vi "FPGA Server.vi"() -> ()   [LabVIEW 2014]
doc: "Accepts inputs from a host based VI for controlling analog and digital outputs on a R-series board containing an FPGA. This VI will produce 4 different signal types dependent on the user input and the channel of interest. When the <B>WaveType</B> is set to laser, the first three channels will produce either a sine or square wave at the frequency <B>f0</B> while the last two produce only square waves. When the wavetype is set to speaker or none, all channels produce the same signal (although for the speaker, signals with a gain of <B>Amp</B> applied)."
uses:
  Utilities/FPGA/Controls/FxdPt Props.ctl
  Reusable/PAS/Main/Controls/Laser Modulation.ctl
  <vilib>/Platform/TimedLoop/XDataNode/timing_clust.ctl
  <vilib>/Platform/TimedLoop/XDataNode/nitl_modes.ctl
  <vilib>/Platform/TimedLoop/XDataNode/wakeup.ctl
  <vilib>/rvi/Emulation/niFpgaGetClockAttributes.vi
  <vilib>/rvi/Emulation/niFpgaSctlEmulationGetInTimedLoop.vi
  <vilib>/rvi/Emulation/niFpgaEmulationReportErrorSimple.vi
  <vilib>/rvi/Emulation/niFpgaProcessEmulError.vi
  <vilib>/rvi/eio/common/nirviEmuTemplateMethod_errors.vi
  <vilib>/rvi/Memory/Memory_Emulation/nirvimemoryFastEmulation.vi
  <vilib>/rvi/Memory/Memory_Emulation/nirvimemoryEmulation.vi
  <vilib>/rvi/Emulation/niFpgaEmulationIsFPGAContextNoSignature.vi
  <vilib>/rvi/DataTransferAndStorage/Container/Common/niFpgaContainerGetUniqueNameForEmu.vi
  <vilib>/rvi/errors/nirviReportUnexpectedCaseInternalError (U32).vi
  <vilib>/rvi/Emulation/niFpgaCriticalErrorInLSC.vi
  <vilib>/rvi/interface/RandomDataEmulation/niFpgaRandomDataHandleErrors.vi
  <vilib>/eio/EIONode/EIONode.xnode
  <vilib>/rvi/DataTransferAndStorage/Container/XNode/niFpgaContainer.xnode
  <vilib>/rvi/FXPMathLib/FxpMul/XNode/nifxpmath_Multiplier.xnode
  <vilib>/rvi/FXPMathLib/FxpAdd/XNode/nifxpmath_Add.xnode
  <vilib>/rvi/interface/RandomDataEmulation/nirviRandomDataFpgaReadWriteTemplate.vi
  <vilib>/Platform/TimedLoop/XDataNode/XDataNode.xnode
  <vilib>/Platform/TimedLoop/XDataNode/XDNodeRunTimeDep.lvlib
  <vilib>/rvi/FXPMathLib/sim/FxpSim.dll
panel:
  out "Direction":bool
  out "error out":errorcluster
  in  "iSpk Enable":T1={"Ch1"=TRUE, "Ch2"=TRUE, "Ch3"=TRUE, "Ch4"=TRUE, "Ch5"=TRUE}
  in  "Speaker":cluster{"Voltage":fxp<+,14,1>, "Offset":i16}
  in  "Spk Enable":bool
  in  "LaserEn":T1
  in  "Cell 5":T2 {"Offset" format="%#.6f"; "Scale" format="%#.6f"}
  in  "Cell 4":T2 {"Offset" format="%#.6f"; "Scale" format="%#.6f"}
  in  "Cell 3":T2 {"Offset" format="%#.6f"; "Scale" format="%#.6f"}
  in  "Cell 2":T2 {"f0" format="%#.6g"; "Offset" format="%#.6f"; "Scale" format="%#.6f"}
  in  "Cell 1":T2 {"f0" format="%.0g"; "Offset" format="%#.6f"; "Scale" format="%#.6f"}
  out "Stopped":bool
  out "SquareOut":T4
  in  "stop":bool
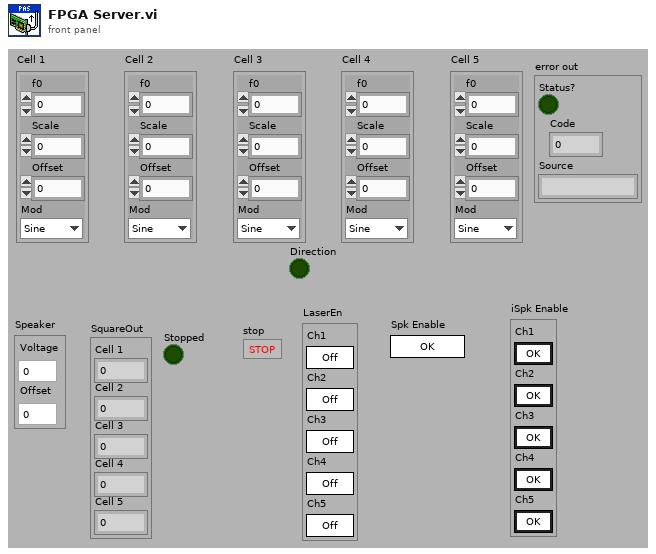
[diagram p1: front panel]
types:
  T1 = cluster{"Ch1":bool, "Ch2":bool, "Ch3":bool, "Ch4":bool, "Ch5":bool}
  T2 = typedef "FxdPt Props.ctl" = cluster{"f0":fxp<+,32,0>, "Scale":fxp<+,14,1>, "Offset":i16, "Mod":T3}
  T3 = typedef "Laser Modulation.ctl" = enum8{"Sine", "Square"}
  T4 = cluster{"Cell 1":i16, "Cell 2":i16, "Cell 3":i16, "Cell 4":i16, "Cell 5":i16}
  T5 = typedef "XDNodeRunTimeDep.lvlib/timing_clust.ctl" = cluster{"Expected End [f-1]":u64, "Actual End [f-1]":u64, "Finished Late? [f-1]":bool, "Expected End [i-1]":u64, "Actual End [i-1]":u64, "Finished Late? [i-1]":bool, "Expected Start [i]":u64, "Actual Start [i]":u64, "Expected Start [f]":u64, "Actual Start [f]":u64, "Source Name":string, "Structure Name":string, "Period":i64, "Deadline":i64, "Offset":i64, "Start":i64, "Priority":i32, "Timeout":i32, "Mode":T6, "Wakeup Reason":T7, "Error":errorcluster, "Source Type":string, "Secondary Source Type":string, "Global End Time":u64, "Global Start Time":u64, "Frame Duration":u64, "Iteration Duration":u64, "Assigned CPU":i32, "I/O Scan Engine Mode":u32}
  T6 = typedef "XDNodeRunTimeDep.lvlib/nitl_modes.ctl" = enum32{"No Change", "Process missed periods, maintain original phase", "Discard missed periods, maintain original phase", "Process missed periods, ignore original phase", "Discard missed periods, ignore original phase"}
  T7 = typedef "XDNodeRunTimeDep.lvlib/wakeup.ctl" = enum32{"Normal", "Aborted", "Asynchronous wakeup", "Timing source error", "Timed loop error", "Timeout"}
  T8 = cluster{"square wave out":i16, "square wave out":i16, "square wave out":i16, "square wave out":i16, "square wave out":i16}
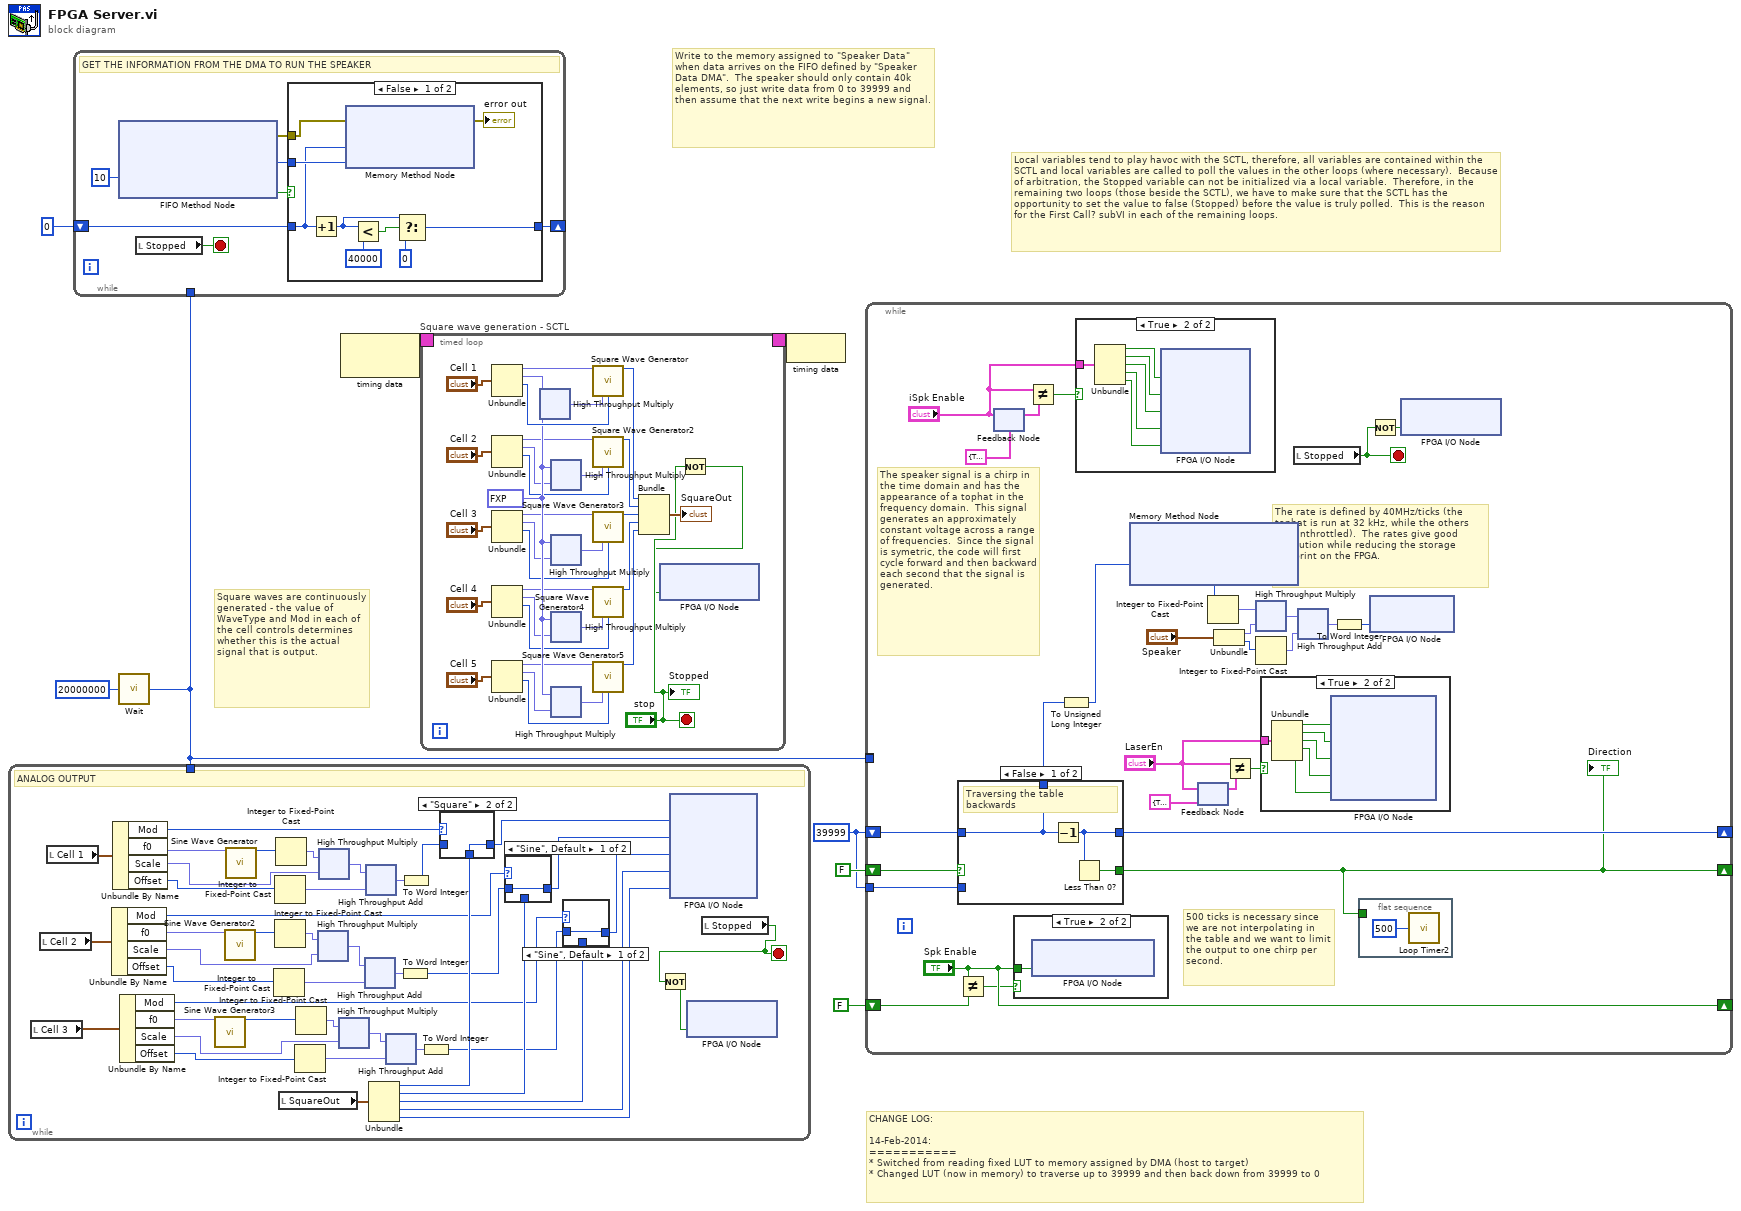
[diagram p0: block diagram]
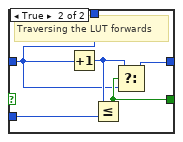
[diagram p6: hidden frame]
diagram:
  w3 = u32 20000000 ("Count(Ticks)")
  w1 = 39999
  # "Write to the memory assigned to \"Speaker Data\" when data arrives on the FIFO defined by \"Speaker Data DMA\".  The speaker should only contain 40k elements, so just write data from 0 to 39999 and then assume that the next write begins a new signal."
  # "CHANGE LOG:\n\n14-Feb-2014:\n===========\n* Switched from reading fixed LUT to memory assigned by DMA (host to target)\n* Changed LUT (now in memory) to traverse up to 39999 and then back down from 39999 to 0"
  # "Square waves are continuously generated - the value of WaveType and Mod in each of the cell controls determines whether this is the actual signal that is output."
  # "Local variables tend to play havoc with the SCTL, therefore, all variables are contained within the SCTL and local variables are called to poll the values in the other loops (where necessary).  Because of arbitration, the Stopped variable can not be initialized via a local variable.  Therefore, in the remaining two loops (those beside the SCTL), we have to make sure that the SCTL has the opportunity to set the value to false (Stopped) before the value is truly polled.  This is the reason for the First Call? subVI in each of the remaining loops."
  n1 = while "Analog Output" {
    tunnel: w3 -> [_]
    stop <- w9 stop-if-true
    # "ANALOG OUTPUT"
    n2 = local read "Cell 3"() -> (w16:T2)
    n3 = local read "Cell 2"() -> (w17:T2)
    n4 = local read "Cell 1"() -> (w18:T2)
    n5 = Unbundle By Name(w17) -> ("Mod"=w11:T3, "f0"=w29:fxp<+,32,0>, "Scale"=w28:fxp<+,14,1>, "Offset"=w27:i16)
    n6 = Unbundle By Name(w18) -> ("Mod"=w12:T3, "f0"=w37:fxp<+,32,0>, "Scale"=w36:fxp<+,14,1>, "Offset"=w35:i16)
    n7 = Unbundle By Name(w16) -> ("Mod"=w10:T3, "f0"=w24:fxp<+,32,0>, "Scale"=w25:fxp<+,14,1>, "Offset"=w26:i16)
    n8 = call "Sine Wave Generator3"("frequency (periods/tick)"=w24) -> ("sine out"=w21:i16)  [unwired: 14 in]
    n9 = call "Sine Wave Generator2"("frequency (periods/tick)"=w29) -> ("sine out"=w32:i16)  [unwired: 14 in]
    n10 = call "Sine Wave Generator"("frequency (periods/tick)"=w37) -> ("sine out"=w40:i16)  [unwired: 14 in]
    n11 = Integer to Fixed-Point Cast(integer=w27) -> (fixed-point=w34:fxp<+/-,16,16>)  [unwired: 1 in]
    n12 = Integer to Fixed-Point Cast(integer=w35) -> (fixed-point=w38:fxp<+/-,16,16>)  [unwired: 1 in]
    n13 = Integer to Fixed-Point Cast(integer=w32) -> (fixed-point=w33:fxp<+/-,16,16>)  [unwired: 1 in]
    n14 = Integer to Fixed-Point Cast(integer=w40) -> (fixed-point=w39:fxp<+/-,16,16>)  [unwired: 1 in]
    n15 = local read "SquareOut"() -> (w46:T4)
    n16 = Integer to Fixed-Point Cast(integer=w26) -> (fixed-point=w19:fxp<+/-,16,16>)  [unwired: 1 in]
    n17 = Integer to Fixed-Point Cast(integer=w21) -> (fixed-point=w20:fxp<+/-,16,16>)  [unwired: 1 in]
    n18 = xnode ("High Throughput Multiply")("x"=w33, "y"=w28) -> ("x*y"=w30:fxp<+/-,30,17>)
    n19 = xnode ("High Throughput Multiply")("x"=w39, "y"=w36) -> ("x*y"=w42:fxp<+/-,30,17>)
    n20 = xnode ("High Throughput Multiply")("x"=w20, "y"=w25) -> ("x*y"=w23:fxp<+/-,30,17>)
    n21 = xnode ("High Throughput Add")("x"=w30, "y"=w34) -> ("x+y"=w31:fxp<+/-,16,16>)
    n22 = xnode ("High Throughput Add")("x"=w42, "y"=w38) -> ("x+y"=w41:fxp<+/-,16,16>)
    n23 = Unbundle(w46) -> ("Cell 1"=w45:i16, "Cell 2"=w44:i16, "Cell 3"=w43:i16, "Cell 4"=w48:i16, "Cell 5"=w47:i16)
    n24 = xnode ("High Throughput Add")("x"=w23, "y"=w19) -> ("x+y"=w22:fxp<+/-,16,16>)
    n25 = To Word Integer(number=w31) -> (16bit integer=w14:i16)
    n26 = To Word Integer(number=w41) -> (16bit integer=w15:i16)
    n27 = To Word Integer(number=w22) -> (16bit integer=w13:i16)
    n28 = case shown="\"Square\"" w12 {
      tunnel: w45 -> [_ w57]
      tunnel: [w56 w57] -> w51
      tunnel: w15 -> [w56 _]
      frame "Sine", Default {
      }
      frame "Square" {
      }
    }
    n29 = case shown="\"Sine\", Default" w11 {
      tunnel: w44 -> [_ w55]
      tunnel: [w54 w55] -> w50
      tunnel: w14 -> [w54 _]
      frame "Sine", Default {
      }
      frame "Square" {
      }
    }
    n30 = case shown="\"Sine\", Default" w10 {
      tunnel: w43 -> [_ w53]
      tunnel: [w52 w53] -> w49
      tunnel: w13 -> [w52 _]
      frame "Sine", Default {
      }
      frame "Square" {
      }
    }
    n31 = xnode "FPGA I/O Node"("Ch 1 AO"=w51, "Ch 2 AO"=w50, "Ch 3 AO"=w49, "Ch 4 AO"=w48, "Ch 5 AO"=w47) -> ()  [unwired: 5 in, 5 out]
    n32 = local read "Stopped"() -> (w9:bool)
    n33 = Not(x=w9) -> (.not. x?=w8:bool)
    n34 = xnode "FPGA I/O Node"("AO Loop"=w8) -> ()  [unwired: 1 in, 1 out]
  }
  n35 = while {
    tunnel: w3 -> [_]
    shift-right: [w59] -> _
    shift-left: u32 0 ("Address") -> [w60]
    stop <- w64 stop-if-true
    # "GET THE INFORMATION FROM THE DMA TO RUN THE SPEAKER"
    n36 = xnode ("FIFO Method Node")("Timeout"=10) -> ("Element"=w62:i16, "Timed Out?"=w61:bool, "error out"=w58:errorcluster)  [unwired: 2 in, 1 out]
    n37 = local read "Stopped"() -> (w64:bool)
    n38 = case shown="False" w61 {
      tunnel: w62 -> [w73 _]
      tunnel: w60 -> [w72 w74]
      tunnel: [w67 w74] -> w59
      tunnel: w58 -> [w66 _]
      frame False {
        n39 = Increment(x=w72) -> (x+1=w69:u32)
        n40 = xnode ("Memory Method Node")("Address"=w72, "Data"=w73, "error in (no error)"=w66) -> ("error out"=→"error out":errorcluster)  [unwired: 1 in, 1 out]
        n41 = Less?(x=w69, y=u32 40000) -> (x < y?=w70:bool)
        n42 = Select(t=w69, s=w70, f=u32 0) -> (s? t:f=w67:u32)
      }
      frame True {
      }
    }
  }
  n43 = call "Wait"("Count(Ticks)"=w3) -> ()  [unwired: 1 out]
  n44 = node-c288() -> (w7:T5)  [unwired: 1 in]
  n45 = timed-loop "Square wave generation - SCTL" {
    timing: w7 -> [_]
    timing-out: [_] -> w6
    stop <- "stop" stop-if-true
    w97 = fxp<+,15,15> 32767.0 ("n")
    n46 = Unbundle("Cell 1") -> ("f0"=w100:fxp<+,32,0>, "Scale"=w99:fxp<+,14,1>, "Offset"=w98:i16)  [unwired: 1 out]
    n47 = Unbundle("Cell 2") -> ("f0"=w88:fxp<+,32,0>, "Scale"=w87:fxp<+,14,1>, "Offset"=w89:i16)  [unwired: 1 out]
    n48 = Unbundle("Cell 3") -> ("f0"=w85:fxp<+,32,0>, "Scale"=w86:fxp<+,14,1>, "Offset"=w90:i16)  [unwired: 1 out]
    n49 = Unbundle("Cell 4") -> ("f0"=w84:fxp<+,32,0>, "Scale"=w83:fxp<+,14,1>, "Offset"=w91:i16)  [unwired: 1 out]
    n50 = Unbundle("Cell 5") -> ("f0"=w78:fxp<+,32,0>, "Scale"=w77:fxp<+,14,1>, "Offset"=w92:i16)  [unwired: 1 out]
    n51 = xnode ("High Throughput Multiply")("x"=w99, "y"=w97) -> ("x*y"=w102:fxp<+,29,16>)
    n52 = xnode ("High Throughput Multiply")("x"=w97, "y"=w87) -> ("x*y"=w80:fxp<+,29,16>)
    n53 = xnode ("High Throughput Multiply")("x"=w97, "y"=w86) -> ("x*y"=w81:fxp<+,29,16>)
    n54 = xnode ("High Throughput Multiply")("x"=w97, "y"=w83) -> ("x*y"=w82:fxp<+,29,16>)
    n55 = xnode ("High Throughput Multiply")("x"=w97, "y"=w77) -> ("x*y"=w79:fxp<+,29,16>)
    n56 = call "Square Wave Generator"("frequency (periods/tick)"=w100, "amplitude"=w102, "offset"=w98) -> ("square wave out"=w108:i16)  [unwired: 12 in]
    n57 = call "Square Wave Generator2"("frequency (periods/tick)"=w88, "amplitude"=w80, "offset"=w89) -> ("square wave out"=w107:i16)  [unwired: 12 in]
    n58 = call "Square Wave Generator3"("frequency (periods/tick)"=w85, "amplitude"=w81, "offset"=w90) -> ("square wave out"=w106:i16)  [unwired: 12 in]
    n59 = call "Square Wave Generator4"("frequency (periods/tick)"=w84, "amplitude"=w82, "offset"=w91) -> ("square wave out"=w105:i16)  [unwired: 12 in]
    n60 = call "Square Wave Generator5"("frequency (periods/tick)"=w78, "amplitude"=w79, "offset"=w92) -> ("square wave out"=w104:i16)  [unwired: 12 in]
    n61 = Bundle("square wave out"=w108, "square wave out"=w107, "square wave out"=w106, "square wave out"=w105, "square wave out"=w104) -> (→"SquareOut":T8)  [unwired: 1 in]
    n62 = Not(x="stop") -> (.not. x?=w75:bool)
    n63 = xnode "FPGA I/O Node"("SQW Loop"=w75) -> ()  [unwired: 1 in, 1 out]
    "Stopped" <- "stop"
  }
  n64 = node-c288(w6) -> ()
  n65 = while {
    shift-right: [w130] -> _
    shift-left: FALSE -> [w140]
    shift-right: [w131] -> _
    shift-left: w1 -> [w132]
    shift-right: ["Spk Enable"] -> _
    shift-left: FALSE ("Spk Enable") -> [w138]
    tunnel: [w123] -> _
    tunnel: w3 -> [w123]
    tunnel: w1 -> [w113]
    stop <- w125 stop-if-true
    # "The rate is defined by 40MHz/ticks (the tophat is run at 32 kHz, while the others are unthrottled).  The rates give good resolution while reducing the storage footprint on the FPGA."
    # "500 ticks is necessary since we are not interpolating in the table and we want to limit the output to one chirp per second."
    # "The speaker signal is a chirp in the time domain and has the appearance of a tophat in the frequency domain.  This signal generates an approximately constant voltage across a range of frequencies.  Since the signal is symetric, the code will first cycle forward and then backward each second that the signal is generated."
    n66 = case "Check where we are in the chirp" shown="False" w140 {
      tunnel: w132 -> [w155 w159]
      tunnel: [w157 w161] -> w130
      tunnel: [w155 w159] -> w112
      tunnel: [w156 w160] -> w131
      tunnel: w113 -> [_ w158]
      frame False {
        # "Traversing the table backwards"
        n67 = Decrement(x=w155) -> (x-1=w156:i32)
        n68 = Less Than 0?(x=w156) -> (x < 0?=w157:bool)
      }
      frame True {
        # "Traversing the LUT forwards"
        n69 = Increment(x=w159) -> (x+1=w162:i32)
        n70 = Less Or Equal?(x=w162, y=w158) -> (x <= y?=w161:bool)
        n71 = Select(t=w162, s=w161, f=w159) -> (s? t:f=w160:i32)
      }
    }
    "Direction" <- w130
    n72 = Not Equal?(x="Spk Enable", y=w138) -> (x != y?=w137:bool)
    n73 = feedback #1(T1 {"Ch1"=TRUE, "Ch2"=TRUE, "Ch3"=TRUE, "Ch4"=TRUE, "Ch5"=TRUE} ("iSpk Enable")) -> (w129:T1)
    n74 = feedback-in #1("iSpk Enable") -> ()
    n75 = case shown="True" w137 {
      tunnel: "Spk Enable" -> [_ w154]
      frame False {
      }
      frame True {
        n76 = xnode "FPGA I/O Node"("Speaker Enable"=w154) -> ()  [unwired: 1 in, 1 out]
      }
    }
    n77 = Not Equal?(x="iSpk Enable", y=w129) -> (x != y?=w127:bool)
    n78 = To Unsigned Long Integer(number=w112) -> (unsigned 32bit integer=w111:u32)
    n79 = case shown="True" w127 {
      tunnel: "iSpk Enable" -> [_ w146]
      frame False {
      }
      frame True {
        n80 = Unbundle(w146) -> ("Ch1"=w145:bool, "Ch2"=w144:bool, "Ch3"=w143:bool, "Ch4"=w142:bool, "Ch5"=w141:bool)
        n81 = xnode "FPGA I/O Node"("Spk Sel 2"=w145, "Spk Sel 1"=w144, "Spk Sel 3"=w143, "Spk Sel 4"=w142, "Spk Sel 5"=w141) -> ()  [unwired: 5 in, 5 out]
      }
    }
    n82 = xnode ("Memory Method Node")("Address"=w111) -> ("Data"=w114:i16)  [unwired: 1 in, 1 out]
    n83 = feedback #2(T1 {"Ch1"=TRUE, "Ch2"=TRUE, "Ch3"=TRUE, "Ch4"=TRUE, "Ch5"=TRUE} ("LaserEn")) -> (w133:T1)
    n84 = feedback-in #2("LaserEn") -> ()
    n85 = Integer to Fixed-Point Cast(integer=w114) -> (fixed-point=w120:fxp<+/-,16,16>)  [unwired: 1 in]
    n86 = Unbundle("Speaker") -> ("Voltage"=w117:fxp<+,14,1>, "Offset"=w116:i16)
    n87 = Not Equal?(x="LaserEn", y=w133) -> (x != y?=w135:bool)
    n88 = xnode ("High Throughput Multiply")("x"=w120, "y"=w117) -> ("x*y"=w122:fxp<+/-,30,17>)
    n89 = Integer to Fixed-Point Cast(integer=w116) -> (fixed-point=w121:fxp<+/-,16,16>)  [unwired: 1 in]
    n90 = case shown="True" w135 {
      tunnel: "LaserEn" -> [_ w153]
      frame False {
      }
      frame True {
        n91 = Unbundle(w153) -> ("Ch1"=w152:bool, "Ch2"=w151:bool, "Ch3"=w150:bool, "Ch4"=w149:bool, "Ch5"=w148:bool)
        n92 = xnode "FPGA I/O Node"("Ch 1 Enable"=w152, "Ch 2 Enable"=w151, "Ch 3 Enable"=w150, "Ch 4 Enable"=w149, "Ch 5 Enable"=w148) -> ()  [unwired: 5 in, 5 out]
      }
    }
    n93 = local read "Stopped"() -> (w125:bool)
    n94 = xnode ("High Throughput Add")("x"=w122, "y"=w121) -> ("x+y"=w118:fxp<+/-,16,16>)
    n95 = To Word Integer(number=w118) -> (16bit integer=w119:i16)
    n96 = flat-sequence {
      tunnel: w130 -> [_]
      frame #0 {
        n97 = call "Loop Timer2"("Count(Ticks)"=u32 500) -> ()  [unwired: 1 out]
      }
    }
    n98 = Not(x=w125) -> (.not. x?=w124:bool)
    n99 = xnode "FPGA I/O Node"("Speaker"=w119) -> ()  [unwired: 1 in, 1 out]
    n100 = xnode "FPGA I/O Node"("Main Loop"=w124) -> ()  [unwired: 1 in, 1 out]
  }
